vi "log analysis_gps.vi"() -> ()   [LabVIEW 2019] (continued)
03*697ae526\n\tsystem status\tnormal 2 28.100000 0 0\trobot status\t219.301877\t108.117218\t8.204700\t-1.556836\t0.092169\t-13.868102\t0.000000\t0.000000\n\t\n15:19:07.8\tlog_raw\tgps_raw\t#DUALANTENNAHEADINGA,USB3,0,49.0,FINESTEERING,2107,281965.800,02008000,d426,15824;SOL_COMPUTED,NARROW_FLOAT,-1.000000000,141.790161133,47.706295013,0.0,360.000000000,180.000000000,\"631T\",19,7,7,7,04,00,20,03*80dc72b9\n\tsystem status\tnormal 2 28.200000 0 0\trobot status\t219.302350\t108.113495\t8.203600\t-1.556726\t0.093605\t-13.864311\t0.000000\t0.000000\n\t\n15:19:08.3\tlog_raw\tgps_raw\t#DUALANTENNAHEADINGA,USB3,0,48.5,FINESTEERING,2107,281966.300,02008000,d426,15824;SOL_COMPUTED,NARROW_FLOAT,-1.000000000,166.037078857,-7.414306641,0.0,293.067352295,180.000000000,\"631T\",18,7,7,7,04,00,20,03*b88985fa\n\tsystem status\tnormal 2 28.200000 0 0\trobot status\t219.302993\t108.111164\t8.202900\t-1.556945\t0.093314\t-13.860391\t0.000000\t0.000000\n\t\n15:19:08.8\tlog_raw\tgps_raw\t#DUALANTENNAHEADINGA,USB3,0,48.5,FINESTEERING,2107,281966.800,02008000,d426,15824;SOL_COMPUTED,NARROW_FLOAT,-1.000000000,165.893447876,-6.919708252,0.0,296.453521729,180.000000000,\"631T\",17,7,7,7,04,00,20,03*8e2fbaf6\n\tsystem status\tnormal 2 28.100000 0 0\trobot status\t219.303827\t108.110162\t8.202400\t-1.557673\t0.092284\t-13.858493\t0.000000\t0.000000\n\t\n15:19:09.3\tlog_raw\tgps_raw\t#DUALANTENNAHEADINGA,USB3,0,48.5,FINESTEERING,2107,281967.300,02008000,d426,15824;SOL_COMPUTED,NARROW_FLOAT,-1.000000000,160.223464966,16.144151688,0.0,238.524597168,180.000000000,\"631T\",17,9,9,9,04,00,20,23*6b3012d0\n\tsystem status\tnormal 2 28.100000 0 0\trobot status\t219.306713\t108.109707\t8.201900\t-1.552890\t0.147275\t-13.759160\t0.122000\t-0.037000\n\t\n15:19:09.8\tlog_raw\tgps_raw\t#DUALANTENNAHEADINGA,USB3,0,48.5,FINESTEERING,2107,281967.800,02008000,d426,15824;SOL_COMPUTED,NARROW_FLOAT,-1.000000000,161.228576660,12.383532524,0.0,230.067184448,180.000000000,\"631T\",17,9,9,9,04,00,20,23*e747bf89\n\tsystem status\tnormal 2 28.100000 0 0\trobot status\t219.452339\t108.074928\t8.203100\t-1.465337\t0.190470\t-13.748043\t0.310000\t-0.019000\n\t\n15:19:10.3\tlog_raw\tgps_raw\t#DUALANTENNAHEADINGA,USB3,0,48.5,FINESTEERING,2107,281968.300,02000000,d426,15824;SOL_COMPUTED,NARROW_FLOAT,-1.000000000,166.146408081,14.704567909,0.0,156.659332275,180.000000000,\"631T\",17,9,9,9,04,00,20,23*68c6ea3a\n\tsystem status\tnormal 2 28.100000 0 0\trobot status\t219.578981\t108.043104\t8.204000\t-1.443728\t0.109997\t-13.833640\t0.283000\t-0.029000\n\t\n15:19:10.8\tlog_raw\tgps_raw\t#DUALANTENNAHEADINGA,USB3,0,48.5,FINESTEERING,2107,281968.800,02000000,d426,15824;SOL_COMPUTED,NARROW_FLOAT,-1.000000000,165.495330811,15.543543816,0.0,158.767318726,180.000000000,\"631T\",20,9,9,9,04,00,20,23*d314ab6c\n\tsystem status\tnormal 2 28.100000 0 0\trobot status\t219.724585\t108.004268\t8.205700\t-1.319380\t-0.022819\t-13.987268\t0.304000\t-0.003000\n\t\n15:19:11.3\tlog_raw\tgps_raw\t#DUALANTENNAHEADINGA,USB3,0,49.0,FINESTEERING,2107,281969.300,02000000,d426,15824;SOL_COMPUTED,NARROW_FLOAT,-1.000000000,139.943130493,-43.141418457,0.0,292.614349365,180.000000000,\"631T\",18,9,9,9,04,00,20,23*245444fd\n\tsystem status\tnormal 2 28.100000 0 0\trobot status\t219.855800\t107.968427\t8.207300\t-1.286734\t-0.015172\t-14.026863\t0.301000\t-0.006000\n\t\n15:19:11.8\tlog_raw\tgps_raw\t#DUALANTENNAHEADINGA,USB3,0,49.0,FINESTEERING,2107,281969.800,02000000,d426,15824;SOL_COMPUTED,NARROW_FLOAT,-1.000000000,140.197708130,-42.675354004,0.0,291.665954590,180.000000000,\"631T\",18,9,9,9,04,00,20,23*76897fdf\n\tsystem status\tnormal 2 28.100000 0 0\trobot status\t219.994546\t107.929885\t8.209200\t-1.297821\t0.001182\t-14.197346\t0.292000\t-0.016000\n\t\n15:19:12.3\tlog_raw\tgps_raw\t#DUALANTENNAHEADINGA,USB3,0,47.0,FINESTEERING,2107,281970.300,02000000,d426,15824;SOL_COMPUTED,NARROW_FLOAT,-1.000000000,136.818527222,-33.589324951,0.0,360.000000000,180.000000000,\"631T\",19,9,9,9,04,00,20,23*7b126b36\n\tsystem status\tnormal 2 28.100000 0 0\trobot status\t220.128217\t107.891100\t8.212500\t-1.413694\t0.161534\t-14.297386\t0.300000\t-0.004000\n\t\n15:19:12.8\tlog_raw\tgps_raw\t#DUALANTENNAHEADINGA,USB3,0,47.0,FINESTEERING,2107,281970.800,02000000,d426,15824;SOL_COMPUTED,NARROW_FLOAT,-1.000000000,136.650482178,-33.009735107,0.0,360.000000000,180.000000000,\"631T\",18,9,9,9,04,00,20,23*68bce87c\n\tsystem status\tnormal 2 28.100000 0 0\trobot status\t220.263771\t107.850315\t8.215700\t-1.551866\t0.293784\t-14.401574\t0.293000\t-0.008000\n\t\n15:19:13.3\tlog_raw\tgps_raw\t#DUALANTENNAHEADINGA,USB3,0,45.5,FINESTEERING,2107,281971.300,02000000,d426,15824;SOL_COMPUTED,NARROW_FLOAT,-1.000000000,137.123779297,-38.778259277,0.0,360.000000000,180.000000000,\"631T\",18,9,9,9,04,00,20,23*afd68441\n\tsystem status\tnormal 2 28.100000 0 0\trobot status\t220.401004\t107.805900\t8.218700\t-1.450367\t0.498611\t-14.556311\t0.301000\t-0.011000\n\t\n15:19:13.8\tlog_raw\tgps_raw\t#DUALANTENNAHEADINGA,USB3,0,45.5,FINESTEERING,2107,281971.800,02000000,d426,15824;SOL_COMPUTED,NARROW_FLOAT,-1.000000000,138.481918335,-40.903717041,0.0,360.000000000,180.000000000,\"631T\",17,7,7,7,04,00,20,03*998ba3b4\n\tsystem status\tnormal 2 28.100000 0 0\trobot status\t220.538888\t107.760543\t8.220800\t-1.387819\t0.562236\t-14.770983\t0.297000\t-0.058000\n\t\n15:19:14.3\tlog_raw\tgps_raw\t#DUALANTENNAHEADINGA,USB3,0,48.5,FINESTEERING,2107,281972.300,02000000,d426,15824;SOL_COMPUTED,NARROW_FLOAT,-1.000000000,122.800582886,-18.535125732,0.0,360.000000000,180.000000000,\"631T\",18,7,7,7,04,00,20,03*a3dfc53a\n\tsystem status\tnormal 2 28.100000 0 0\trobot status\t220.684115\t107.713725\t8.225400\t-1.489746\t0.729168\t-15.149259\t0.323000\t-0.019000\n\t\n15:19:14.8\tlog_raw\tgps_raw\t#DUALANTENNAHEADINGA,USB3,0,48.5,FINESTEERING,2107,281972.800,02000000,d426,15824;SOL_COMPUTED,NARROW_FLOAT,-1.000000000,124.024436951,-18.181030273,0.0,360.000000000,180.000000000,\"631T\",19,7,7,7,04,00,20,03*7aaae106\n\tsystem status\tnormal 2 28.000000 0 0\trobot status\t220.823247\t107.667621\t8.231100\t-1.707730\t0.719198\t-15.929117\t0.256000\t-0.109000\n\t\n15:19:15.3\tlog_raw\tgps_raw\t#DUALANTENNAHEADINGA,USB3,0,47.5,FINESTEERING,2107,281973.300,02000000,d426,15824;SOL_COMPUTED,NARROW_FLOAT,-1.000000000,122.042884827,-22.737487793,0.0,360.000000000,180.000000000,\"631T\",19,7,7,7,04,00,20,03*1f55fb10\n\tsystem status\tnormal 2 28.000000 0 0\trobot status\t220.956067\t107.616714\t8.234300\t-1.546838\t0.621611\t-17.048894\t0.328000\t-0.004000\n\t\n15:19:15.8\tlog_raw\tgps_raw\t#DUALANTENNAHEADINGA,USB3,0,47.5,FINESTEERING,2107,281973.800,02000000,d426,15824;SOL_COMPUTED,NARROW_FLOAT,-1.000000000,123.718307495,-22.855773926,0.0,360.000000000,180.000000000,\"631T\",19,7,7,7,04,00,20,03*d5b1223e\n\tsystem status\tnormal 2 27.800000 0 0\trobot status\t221.089499\t107.561166\t8.235900\t-1.404373\t0.484391\t-18.472087\t0.229000\t-0.159000\n\t\n15:19:16.3\tlog_raw\tgps_raw\t#DUALANTENNAHEADINGA,USB3,0,47.5,FINESTEERING,2107,281974.300,02000000,d426,15824;SOL_COMPUTED,NARROW_FLOAT,-1.000000000,126.303939819,-25.588958740,0.0,360.000000000,180.000000000,\"631T\",20,7,7,7,04,00,20,03*39a380db\n\tsystem status\tnormal 2 27.800000 0 0\trobot status\t221.221746\t107.503167\t8.238200\t-1.480054\t0.670255\t-19.868861\t0.268000\t-0.096000\n\t\n15:19:16.8\tlog_raw\tgps_raw\t\tsystem status\tnormal 2 27.800000 0 0\trobot status\t221.353565\t107.442341\t8.242100\t-1.646339\t0.593532\t-21.133921\t0.306000\t-0.008000\n\t\n15:19:17.3\tlog_raw\tgps_raw\t\tsystem status\tnormal 2 28.000000 0 0\trobot status\t221.483986\t107.376940\t8.246600\t-1.582498\t0.515204\t-22.081277\t0.288000\t-0.060000\n\t\n15:19:17.8\tlog_raw\tgps_raw\t\tsystem status\tnormal 2 28.000000 0 0\trobot status\t221.610837\t107.309899\t8.249600\t-1.462249\t0.554475\t-22.719176\t0.412000\t0.141000\n\t\n15:19:18.3\tlog_raw\tgps_raw\t\tsystem status\tnormal 2 28.100000 0 0\trobot status\t221.736004\t107.242196\t8.251300\t-1.432747\t0.573608\t-23.074714\t0.316000\t0.037000\n\t\n15:19:18.8\tlog_raw\tgps_raw\t\tsystem status\tnormal 2 28.100000 0 0\trobot status\t221.859914\t107.174246\t8.252600\t-1.427237\t0.406480\t-23.239314\t0.289000\t0.008000\n\t\n15:19:19.3\tlog_raw\tgps_raw\t#INSPVAXA,USB3,0,49.5,FINESTEERING,2107,281977.350,02008000,471d,15824;INS_ALIGNMENT_COMPLETE,INS_RTKFIXED,37.37109525402,126.72334121062,8.2543,22.3000,-0.1170,0.2421,0.0133,-1.435832187,0.337185774,113.410271664,0.3981,0.2933,0.5166,0.1081,0.0923,0.0755,0.1541,0.1553,4.9775,0f000001,0*5c2d119f\n\tsystem status\tnormal 2 28.100000 0 0\trobot status\t221.986722\t107.103576\t8.254300\t-1.435832\t0.337186\t-23.410272\t0.294000\t0.028000\n\t\n15:19:19.8\tlog_raw\tgps_raw\t\tsystem status\tnormal 2 28.100000 0 0\trobot status\t222.097089\t107.042706\t8.257000\t-1.370753\t0.338842\t-23.399913\t0.298000\t0.032000\n\t\n15:19:20.3\tlog_raw\tgps_raw\t\tsystem status\tnormal 2 28.100000 0 0\trobot status\t222.231985\t106.969531\t8.259800\t-1.288256\t0.476149\t-23.360701\t0.319000\t0.022000\n\t\n15:19:20.8\tlog_raw\tgps_raw\t#DUALANTENNAHEADINGA,USB3,0,47.5,FINESTEERING,2107,281978.800,02008000,d426,15824;SOL_COMPUTED,NARROW_FLOAT,-1.000000000,98.850494385,15.051933289,0.0,360.000000000,180.000000000,\"631T\",20,7,7,7,04,00,20,03*20b61e65\n\tsystem status\tnormal 2 28.000000 0 0\trobot status\t222.361467\t106.898858\t8.261700\t-1.138019\t0.411063\t-23.031329\t0.236000\t0.133000\n\t\n15:19:21.3\tlog_raw\tgps_raw\t#INSPVAXA,USB3,0,49.0,FINESTEERING,2107,281979.350,02008000,471d,15824;INS_ALIGNMENT_COMPLETE,INS_RTKFIXED,37.37109277757,126.72334695019,8.2625,22.3000,-0.1363,0.2541,0.0099,-1.083954396,0.543239164,111.989343761,0.3985,0.2934,0.5159,0.1083,0.0925,0.0755,0.1539,0.1552,4.9769,0f000001,0*5af8ae3d\n\tsystem status\tnormal 2 27.900000 0 0\trobot status\t222.495124\t106.828715\t8.262500\t-1.083954\t0.543239\t-21.989344\t0.244000\t0.133000\n\t\n15:19:21.8\tlog_raw\tgps_raw\t#INSPVAXA,USB3,0,49.0,FINESTEERING,2107,281979.850,02008000,471d,15824;INS_ALIGNMENT_COMPLETE,INS_RTKFIXED,37.37109223488,126.72334834985,8.2645,22.3000,-0.1140,0.2510,0.0288,-1.130767744,0.597027739,110.592195970,0.3985,0.2934,0.5159,0.1083,0.0925,0.0755,0.1539,0.1552,4.9769,0f000001,0*c15e5176\n\tsystem status\tnormal 2 27.700000 0 0\trobot status\t222.619104\t106.768481\t8.264500\t-1.130768\t0.597028\t-20.592196\t0.292000\t0.067000\n\t\n15:19:22.3\tlog_raw\tgps_raw\t#INSPVAXA,USB3,0,47.5,FINESTEERING,2107,281980.350,02008000,471d,15824;INS_ALIGNMENT_COMPLETE,INS_RTKFIXED,37.37109170650,126.72334980236,8.2673,22.3000,-0.1001,0.2682,0.0069,-1.052775412,0.394834904,108.778696674,0.3992,0.2936,0.5159,0.1082,0.0924,0.0755,0.1537,0.1552,4.9781,0f000001,0*7c12e27f\n\tsystem status\tnormal 2 27.500000 0 0\trobot status\t222.747765\t106.709836\t8.267300\t-1.052775\t0.394835\t-18.778697\t0.298000\t0.063000\n\t\n15:19:22.8\tlog_raw\tgps_raw\t\tsystem status\tnormal 2 27.500000 0 0\trobot status\t222.863745\t106.660014\t8.268600\t-0.838461\t0.276001\t-16.977261\t0.297000\t0.053000\n\t\n15:19:23.3\tlog_raw\tgps_raw\t\tsystem status\tnormal 2 27.600000 4 0\trobot status\t222.994027\t106.612485\t8.270800\t-0.856834\t0.314980\t-15.099494\t0.306000\t0.063000\n\t\n15:19:23.8\tlog_raw\tgps_raw\t#DUALANTENNAHEADINGA,USB3,0,47.5,FINESTEERING,2107,281981.800,02000000,d426,15824;SOL_COMPUTED,NARROW_FLOAT,-1.000000000,85.660850525,58.330966949,0.0,360.000000000,180.000000000,\"631T\",21,7,7,7,04,00,20,03*4d1d89aa\n\tsystem status\tnormal 2 27.600000 4 0\trobot status\t223.126606\t106.570431\t8.273400\t-0.931607\t0.502901\t-13.314554\t0.308000\t0.043000\n\t\n15:19:24.3\tlog_raw\tgps_raw\t#DUALANTENNAHEADINGA,USB3,0,50.0,FINESTEERING,2107,281982.300,02000000,d426,15824;SOL_COMPUTED,NARROW_FLOAT,-1.000000000,91.491950989,60.466197968,0.0,360.000000000,180.000000000,\"631T\",20,7,7,7,04,00,20,03*c36635f4\n\tsystem status\tnormal 2 27.700000 0 0\trobot status\t223.261861\t106.529900\t8.275300\t-0.949553\t0.583973\t-11.945884\t0.297000\t0.040000\n\t\n15:19:24.8\tlog_raw\tgps_raw\t#INSPVAXA,USB3,0,50.0,FINESTEERING,2107,281982.850,02000000,471d,15824;INS_ALIGNMENT_COMPLETE,INS_RTKFIXED,37.37108972334,126.72335727408,8.2765,22.3000,-0.0719,0.2745,0.0019,-0.882780999,0.621145349,100.706035847,0.4014,0.2941,0.5170,0.1080,0.0922,0.0756,0.1534,0.1551,4.9808,0f000001,0*8125501e\n\tsystem status\tnormal 2 27.800000 0 0\trobot status\t223.409597\t106.489718\t8.276500\t-0.882781\t0.621145\t-10.706036\t0.293000\t0.023000\n\t\n15:19:25.3\tlog_raw\tgps_raw\t#INSPVAXA,USB3,0,50.0,FINESTEERING,2107,281983.350,02000000,471d,15824;INS_ALIGNMENT_COMPLETE,INS_RTKFIXED,37.37108941060,126.72335884904,8.2775,22.3000,-0.0682,0.2732,0.0044,-0.923445241,0.570606405,99.817736396,0.4009,0.2937,0.5167,0.1077,0.0921,0.0755,0.1533,0.1550,4.9813,0f000001,0*fb321f29\n\tsystem status\tnormal 2 27.800000 0 0\trobot status\t223.549105\t106.455005\t8.277500\t-0.923445\t0.570606\t-9.817736\t0.249000\t0.097000\n\t\n15:19:25.8\tlog_raw\tgps_raw\t#DUALANTENNAHEADINGA,USB3,0,50.0,FINESTEERING,2107,281983.800,02000000,d426,15824;SOL_COMPUTED,NARROW_FLOAT,-1.000000000,171.677200317,69.382904053,0.0,261.160797119,118.765472412,\"631T\",16,7,7,7,04,00,20,03*68664d6e\n\tsystem status\tnormal 2 27.900000 0 0\trobot status\t223.673813\t106.423577\t8.278600\t-0.753862\t0.396065\t-9.286254\t0.221000\t0.059000\n\t\n15:19:26.3\tlog_raw\tgps_raw\t\tsystem status\tnormal 2 28.100000 0 0\trobot status\t223.691032\t106.410286\t8.277000\t-0.784481\t0.395097\t-9.504168\t0.001000\t0.000000\n\t\n15:19:26.8\tlog_raw\tgps_raw\t#DUALANTENNAHEADINGA,USB3,0,49.0,FINESTEERING,2107,281984.800,02000000,d426,15824;SOL_COMPUTED,NARROW_FLOAT,-1.000000000,180.068710327,69.173255920,0.0,191.709030151,111.731857300,\"631T\",18,7,7,7,04,00,20,03*3faf2cde\n\tsystem status\tnormal 2 28.100000 0 0\trobot status\t223.690316\t106.399747\t8.275200\t-0.784448\t0.393746\t-9.515483\t0.000000\t0.000000\n\t\n15:19:27.3\tlog_raw\tgps_raw\t#INSPVAXA,USB3,0,51.5,FINESTEERING,2107,281985.350,02000000,471d,15824;INS_ALIGNMENT_COMPLETE,INS_RTKFIXED,37.37108883978,126.72336045763,8.2740,22.3000,-0.0197,0.0054,0.0046,-0.783405555,0.390647361,99.517937429,0.4021,0.2930,0.5155,0.1100,0.0923,0.0753,0.1532,0.1549,4.9767,0f000001,0*248bca7d\n\tsystem status\tnormal 2 28.100000 0 0\trobot status\t223.691591\t106.391649\t8.274000\t-0.783406\t0.390647\t-9.517937\t0.000000\t0.000000\n\t\n15:19:27.8\tlog_raw\tgps_raw\t#INSPVAXA,USB3,0,51.5,FINESTEERING,2107,281985.850,02000000,471d,15824;INS_ALIGNMENT_COMPLETE,INS_RTKFIXED,37.37108879564,126.72336048903,8.2732,22.3000,-0.0176,0.0072,0.0041,-0.785106816,0.393235507,99.515755196,0.4021,0.2930,0.5155,0.1100,0.0923,0.0753,0.1532,0.1549,4.9767,0f000001,0*274b58cf\n\tsystem status\tnormal 2 28.100000 0 0\trobot status\t223.694372\t106.386750\t8.273200\t-0.785107\t0.393236\t-9.515755\t0.000000\t0.000000\n\t\n15:19:28.3\tlog_raw\tgps_raw\t#INSPVAXA,USB3,0,48.0,FINESTEERING,2107,281986.350,02000000,471d,15824;INS_ALIGNMENT_COMPLETE,INS_RTKFIXED,37.37108876739,126.72336052169,8.2716,22.3000,-0.0165,0.0095,0.0036,-0.784401118,0.395223207,99.515202134,0.4035,0.2929,0.5152,0.1096,0.0926,0.0753,0.1533,0.1548,4.9684,0f000001,0*a346e64c\n\tsystem status\tnormal 2 28.100000 0 0\trobot status\t223.697265\t106.383614\t8.271600\t-0.784401\t0.395223\t-9.515202\t0.000000\t0.000000\n\t\n15:19:28.8\tlog_raw\tgps_raw\t#INSPVAXA,USB3,0,48.0,FINESTEERING,2107,281986.850,02000000,471d,15824;INS_ALIGNMENT_COMPLETE,INS_RTKFIXED,37.37108874345,126.72336056234,8.2697,22.3000,-0.0165,0.0121,0.0038,-0.783492402,0.394489755,99.515268090,0.4035,0.2929,0.5152,0.1096,0.0926,0.0753,0.1533,0.1548,4.9684,0f000001,0*d15eefc4\n\tsystem status\tnormal 2 28.100000 0 0\trobot status\t223.700866\t106.380957\t8.269700\t-0.783492\t0.394490\t-9.515268\t0.000000\t0.000000\n\t\n15:19:29.3\tlog_raw\tgps_raw\t\tsystem status\tnormal 2 28.000000 0 0\trobot status\t223.744232\t106.373691\t8.270100\t-0.798843\t0.520000\t-9.359082\t0.297000\t-0.003000\n\t\n15:19:29.8\tlog_raw\tgps_raw\t\tsystem status\tnormal 2 28.100000 0 0\trobot status\t223.909115\t106.346672\t8.272000\t-0.747510\t0.256715\t-9.615742\t0.328000\t-0.055000\n\t\n15:19:30.3\tlog_raw\tgps_raw\t\tsystem status\tnormal 2 28.100000 0 0\trobot status\t224.051089\t106.323073\t8.274200\t-0.894303\t0.217307\t-9.628486\t0.311000\t-0.011000\n\t\n15:19:30.8\tlog_raw\tgps_raw\t#INSPVAXA,USB3,0,47.5,FINESTEERING,2107,281988.850,02000000,471d,15824;INS_ALIGNMENT_COMPLETE,INS_RTKFIXED,37.37108797326,126.72336627998,8.2767,22.3000,-0.0630,0.2990,0.0131,-1.082198945,0.183813421,99.716659847,0.4039,0.2931,0.5146,0.1091,0.0928,0.0753,0.1533,0.1544,4.9498,0f000001,0*73d74fed\n\tsystem status\tnormal 2 28.100000 0 0\trobot status\t224.207325\t106.295465\t8.276700\t-1.082199\t0.183813\t-9.716660\t0.302000\t-0.009000\n\t\n15:19:31.3\tlog_raw\tgps_raw\t#INSPVAXA,USB3,0,47.5,FINESTEERING,2107,281989.350,02000000,471d,15824;INS_ALIGNMENT_COMPLETE,INS_RTKFIXED,37.37108771760,126.72336784946,8.2786,22.3000,-0.0596,0.2938,0.0092,-0.873489656,0.138919963,99.763055093,0.4016,0.2938,0.5156,0.1102,0.0931,0.0754,0.1533,0.1542,4.9496,0f000001,0*cc44b012\n\tsystem status\tnormal 2 28.100000 0 0\trobot status\t224.346347\t106.267087\t8.278600\t-0.873490\t0.138920\t-9.763055\t0.292000\t0.011000\n\t\n15:19:31.8\tlog_raw\tgps_raw\t\tsystem status\tnormal 2 28.100000 0 0\trobot status\t224.485443\t106.239017\t8.280100\t-0.782767\t-0.017640\t-9.679057\t0.297000\t0.017000\n\t\n15:19:32.3\tlog_raw\tgps_raw\t\tsystem status\tnormal 2 28.000000 0 0\trobot status\t224.626651\t106.210499\t8.281900\t-0.769512\t0.068077\t-9.236097\t0.360000\t-0.076000\n\t\n15:19:32.8\tlog_raw\tgps_raw\t#INSPVAXA,USB3,0,48.0,FINESTEERING,2107,281990.850,02000000,471d,15824;INS_ALIGNMENT_COMPLETE,INS_RTKFIXED,37.37108694002,126.72337277307,8.2855,22.3000,-0.0481,0.3030,0.0049,-0.965496149,0.214981023,98.709278858,0.4041,0.2964,0.5214,0.1116,0.0937,0.0758,0.1533,0.1541,4.9510,0f000001,0*3e871dfa\n\tsystem status\tnormal 2 28.000000 0 0\trobot status\t224.782473\t106.180775\t8.285500\t-0.965496\t0.214981\t-8.709279\t0.336000\t-0.030000\n\t\n15:19:33.3\tlog_raw\tgps_raw\t#INSPVAXA,USB3,0,49.5,FINESTEERING,2107,281991.350,02000000,471d,15824;INS_ALIGNMENT_COMPLETE,INS_RTKFIXED,37.37108669886,126.72337439108,8.2873,22.3000,-0.0502,0.3004,0.0017,-1.174650007,0.215279567,98.185602057,0.4065,0.2980,0.5270,0.1121,0.0939,0.0762,0.1533,0.1539,4.9506,0f000001,0*29bf6a14\n\tsystem status\tnormal 2 28.000000 0 0\trobot status\t224.925793\t106.154006\t8.287300\t-1.174650\t0.215280\t-8.185602\t0.248000\t0.089000\n\t\n15:19:33.8\tlog_raw\tgps_raw\t\tsystem status\tnormal 2 28.000000 0 0\trobot status\t225.055464\t106.128832\t8.288900\t-1.106111\t0.185902\t-7.711529\t0.340000\t-0.056000\n\t\n15:19:34.3\tlog_raw\tgps_raw\t#INSPVAXA,USB3,0,48.5,FINESTEERING,2107,281992.350,02008000,471d,15824;INS_ALIGNMENT_COMPLETE,INS_RTKFIXED,37.37108621097,126.72337762308,8.2906,22.3000,-0.0509,0.3067,0.0077,-1.111919380,0.301360235,97.469482841,0.4135,0.2993,0.5341,0.1130,0.0941,0.0766,0.1532,0.1538,4.9480,0f000001,0*f7c4fc4c\n\tsystem status\tnormal 2 28.000000 0 0\trobot status\t225.212079\t106.099851\t8.290600\t-1.111919\t0.301360\t-7.469483\t0.444000\t-0.212000\n\t\n15:19:34.8\tlog_raw\tgps_raw\t#INSPVAXA,USB3,0,48.5,FINESTEERING,2107,281992.850,02008000,471d,15824;INS_ALIGNMENT_COMPLETE,INS_RTKFIXED,37.37108597752,126.72337923306,8.2930,22.3000,-0.0486,0.3061,0.0133,-1.174980887,0.150326123,97.387759398,0.4135,0.2993,0.5341,0.1130,0.0941,0.0766,0.1532,0.1538,4.9480,0f000001,0*c1faa1b5\n\tsystem status\tnormal 2 28.000000 0 0\trobot status\t225.354688\t106.073937\t8.293000\t-1.174981\t0.150326\t-7.387759\t0.359000\t-0.095000\n\t\n15:19:35.3\tlog_raw\tgps_raw\t#INSPVAXA,USB3,0,46.0,FINESTEERING,2107,281993.350,02008000,471d,15824;INS_ALIGNMENT_COMPLETE,INS_RTKFIXED,37.37108573998,126.72338082832,8.2949,22.3000,-0.0500,0.2978,0.0061,-1.421543632,0.145972145,97.447075083,0.4166,0.2999,0.5394,0.1132,0.0941,0.0768,0.1531,0.1535,4.9437,0f000001,0*17ed31ac\n\tsystem status\tnormal 2 28.100000 0 0\trobot status\t225.495993\t106.047570\t8.294900\t-1.421544\t0.145972\t-7.447075\t0.251000\t0.057000\n\t\n15:19:35.8\tlog_raw\tgps_raw\t#INSPVAXA,USB3,0,46.0,FINESTEERING,2107,281993.850,02008000,471d,15824;INS_ALIGNMENT_COMPLETE,INS_RTKFIXED,37.37108548434,126.72338234457,8.2959,22.3000,-0.0500,0.2833,0.0078,-1.457872405,0.272327462,97.575825981,0.4166,0.2999,0.5394,0.1132,0.0941,0.0768,0.1531,0.1535,4.9437,0f000001,0*5caa60c3\n\tsystem status\tnormal 2 28.100000 0 0\trobot status\t225.630300\t106.019194\t8.295900\t-1.457872\t0.272327\t-7.575826\t0.294000\t-0.026000\n\t\n15:19:36.3\tlog_raw\tgps_raw\t\tsystem status\tnormal 2 28.100000 0 0\trobot status\t225.748467\t105.992775\t8.298600\t-1.403323\t0.357170\t-7.675488\t0.298000\t-0.031000\n\t\n15:19:36.8\tlog_raw\tgps_raw\t#INSPVAXA,USB3,0,49.0,FINESTEERING,2107,281994.850,02008000,471d,15824;INS_ALIGNMENT_COMPLETE,INS_RTKFIXED,37.37108494308,126.72338542204,8.3016,22.3000,-0.0524,0.2963,0.0111,-1.327091398,0.262905229,97.908015700,0.4162,0.2999,0.5423,0.1120,0.0939,0.0768,0.1530,0.1531,4.9380,0f000001,0*42f9b06f\n\tsystem status\tnormal 2 28.100000 0 0\trobot status\t225.902898\t105.959116\t8.301600\t-1.327091\t0.262905\t-7.908016\t0.294000\t-0.034000\n\t\n15:19:37.3\tlog_raw\tgps_raw\t#INSPVAXA,USB3,0,47.5,FINESTEERING,2107,281995.350,02008000,471d,15824;INS_ALIGNMENT_COMPLETE,INS_RTKFIXED,37.37108466032,126.72338706837,8.3039,22.3000,-0.0576,0.3333,-0.0065,-1.460342907,0.308573578,98.178770776,0.4137,0.2991,0.5422,0.1112,0.0936,0.0766,0.1529,0.1527,4.9332,0f000001,0*ae64a2a4\n\tsystem status\tnormal 2 28.100000 0 0\trobot status\t226.048727\t105.927730\t8.303900\t-1.460343\t0.308574\t-8.178771\t0.301000\t-0.034000\n\t\n15:19:37.8\tlog_raw\tgps_raw\t#INSPVAXA,USB3,0,47.5,FINESTEERING,2107,281995.850,02008000,471d,15824;INS_ALIGNMENT_COMPLETE,INS_RTKFIXED,37.37108438124,126.72338871075,8.3072,22.3000,-0.0531,0.3233,-0.0006,-1.819145416,0.336322767,98.552237530,0.4137,0.2991,0.5422,0.1112,0.0936,0.0766,0.1529,0.1527,4.9332,0f000001,0*cbb88409\n\tsystem status\tnormal 2 28.100000 0 0\trobot status\t226.194206\t105.896752\t8.307200\t-1.819145\t0.336323\t-8.552238\t0.312000\t-0.021000\n\t\n15:19:38.3\tlog_raw\tgps_raw\t#INSPVAXA,USB3,0,47.5,FINESTEERING,2107,281996.350,02000000,471d,15824;INS_ALIGNMENT_COMPLETE,INS_RTKFIXED,37.37108408170,126.72339032288,8.3123,22.3000,-0.0750,0.3139,0.0177,-1.695760628,0.287982482,99.034005489,0.4135,0.2988,0.5426,0.1109,0.0935,0.0765,0.1528,0.1525,4.9294,0f000001,0*c8ba75d6\n\tsystem status\tnormal 2 28.100000 0 0\trobot status\t226.337006\t105.863504\t8.312300\t-1.695761\t0.287982\t-9.034005\t0.263000\t-0.087000\n\t\n15:19:38.8\tlog_raw\tgps_raw\t#INSPVAXA,USB3,0,47.5,FINESTEERING,2107,281996.850,02000000,471d,15824;INS_ALIGNMENT_COMPLETE,INS_RTKFIXED,37.37108376936,126.72339189832,8.3173,22.3000,-0.0870,0.3015,0.0104,-1.544598209,0.423694709,99.865488428,0.4135,0.2988,0.5426,0.1109,0.0935,0.0765,0.1528,0.1525,4.9294,0f000001,0*decac9b0\n\tsystem status\tnormal 2 28.000000 0 0\trobot status\t226.476556\t105.828835\t8.317300\t-1.544598\t0.423695\t-9.865488\t0.314000\t-0.012000\n\t\n15:19:39.3\tlog_raw\tgps_raw\t#INSPVAXA,USB3,0,47.0,FINESTEERING,2107,281997.350,02000000,471d,15824;INS_ALIGNMENT_COMPLETE,INS_RTKFIXED,37.37108342179,126.72339342311,8.3197,22.3000,-0.0655,0.2686,0.0098,-1.474135417,0.714052944,100.935237660,0.4109,0.2981,0.5411,0.1099,0.0931,0.0764,0.1526,0.1523,4.9264,0f000001,0*027bf543\n\tsystem status\tnormal 2 28.000000 0 0\trobot status\t226.611619\t105.790257\t8.319700\t-1.474135\t0.714053\t-10.935238\t0.298000\t-0.044000\n\t\n15:19:39.8\tlog_raw\tgps_raw\t#INSPVAXA,USB3,0,47.0,FINESTEERING,2107,281997.850,02000000,471d,15824;INS_ALIGNMENT_COMPLETE,INS_RTKFIXED,37.37108303856,126.72339495769,8.3212,22.3000,-0.0845,0.2926,0.0185,-1.495781982,0.741465354,102.154050788,0.4109,0.2981,0.5411,0.1099,0.0931,0.0764,0.1526,0.1523,4.9264,0f000001,0*92cd812c\n\tsystem status\tnormal 2 27.800000 0 0\trobot status\t226.747550\t105.747720\t8.321200\t-1.495782\t0.741465\t-12.154051\t0.325000\t-0.013000\n\t\n15:19:40.3\tlog_raw\tgps_raw\t#DUALANTENNAHEADINGA,USB3,0,46.5,FINESTEERING,2107,281998.300,02000000,d426,15824;SOL_COMPUTED,NARROW_FLOAT,-1.000000000,172.084686279,54.228965759,0.0,275.366882324,180.000000000,\"631T\",18,9,9,9,04,00,20,23*6c4f8940\n\tsystem status\tnormal 2 27.800000 0 0\trobot status\t226.869310\t105.708063\t8.323600\t-1.489847\t0.680798\t-13.305228\t0.285000\t-0.048000\n\t\n15:19:40.8\tlog_raw\tgps_raw\t#INSPVAXA,USB3,0,46.5,FINESTEERING,2107,281998.850,02000000,471d,15824;INS_ALIGNMENT_COMPLETE,INS_RTKFIXED,37.37108222334,126.72339800305,8.3261,22.3000,-0.1005,0.2888,0.0175,-1.549699637,0.826090686,104.570528927,0.4090,0.2977,0.5394,0.1094,0.0929,0.0762,0.1525,0.1522,4.9251,0f000001,0*19ed46e2\n\tsystem status\tnormal 2 27.900000 0 0\trobot status\t227.017303\t105.657236\t8.326100\t-1.549700\t0.826091\t-14.570529\t0.291000\t-0.041000\n\t\n15:19:41.3\tlog_raw\tgps_raw\t#INSPVAXA,USB3,0,46.5,FINESTEERING,2107,281999.350,02000000,471d,15824;INS_ALIGNMENT_COMPLETE,INS_RTKFIXED,37.37108175635,126.72339952041,8.3297,22.3000,-0.1125,0.3020,0.0389,-1.388953063,0.939960250,105.504121807,0.4075,0.2973,0.5375,0.1091,0.0928,0.0761,0.1524,0.1521,4.9251,0f000001,0*0f043892\n\tsystem status\tnormal 2 27.900000 0 0\trobot status\t227.151708\t105.605404\t8.329700\t-1.388953\t0.939960\t-15.504122\t0.320000\t0.005000\n\t\n15:19:41.8\tlog_raw\tgps_raw\t#INSPVAXA,USB3,0,46.5,FINESTEERING,2107,281999.850,02000000,471d,15824;INS_ALIGNMENT_COMPLETE,INS_RTKFIXED,37.37108126318,126.72340101598,8.3324,22.3000,-0.1208,0.2855,0.0176,-1.235609650,1.001617450,106.317928452,0.4075,0.2973,0.5375,0.1091,0.0928,0.0761,0.1524,0.1521,4.9251,0f000001,0*a366704e\n\tsystem status\tnormal 2 28.000000 0 0\trobot status\t227.284183\t105.550666\t8.332400\t-1.235610\t1.001617\t-16.317928\t0.353000\t0.073000\n\t\n15:19:42.3\tlog_raw\tgps_raw\t#INSPVAXA,USB3,0,45.5,FINESTEERING,2107,282000.350,02000000,471d,15824;INS_ALIGNMENT_COMPLETE,INS_RTKFIXED,37.37108078810,126.72340249141,8.3350,22.3000,-0.1085,0.2765,0.0052,-1.369966017,1.132397768,106.939829870,0.4067,0.2969,0.5359,0.1090,0.0927,0.0761,0.1523,0.1521,4.9261,0f000001,0*76e4d7c9\n\tsystem status\tnormal 2 28.000000 0 0\trobot status\t227.414874\t105.497936\t8.335000\t-1.369966\t1.132398\t-16.939830\t0.348000\t0.059000\n\t\n15:19:42.8\tlog_raw\tgps_raw\t#INSPVAXA,USB3,0,45.5,FINESTEERING,2107,282000.850,02000000,471d,15824;INS_ALIGNMENT_COMPLETE,INS_RTKFIXED,37.37108030098,126.72340396380,8.3376,22.3000,-0.1078,0.2732,0.0027,-1.376343983,1.101027936,107.303720735,0.4067,0.2969,0.5359,0.1090,0.0927,0.0761,0.1523,0.1521,4.9261,0f000001,0*d0ca4e8b\n\tsystem status\tnormal 2 28.000000 0 0\trobot status\t227.545296\t105.443869\t8.337600\t-1.376344\t1.101028\t-17.303721\t0.357000\t0.093000\n\t\n15:19:43.3\tlog_raw\tgps_raw\t#INSPVAXA,USB3,0,48.0,FINESTEERING,2107,282001.350,02000000,471d,15824;INS_ALIGNMENT_COMPLETE,INS_RTKFIXED,37.37107981419,126.72340544381,8.3410,22.3000,-0.1015,0.2654,0.0098,-1.448342313,0.934631006,107.625890193,0.4067,0.2967,0.5346,0.1090,0.0928,0.0761,0.1522,0.1521,4.9276,0f000001,0*0452f07a\n\tsystem status\tnormal 2 28.100000 0 0\trobot status\t227.676393\t105.389840\t8.341000\t-1.448342\t0.934631\t-17.625890\t0.248000\t-0.063000\n\t\n15:19:43.8\tlog_raw\tgps_raw\t#INSPVAXA,USB3,0,48.0,FINESTEERING,2107,282001.850,02000000,471d,15824;INS_ALIGNMENT_COMPLETE,INS_RTKFIXED,37.37107932053,126.72340689230,8.3455,22.3000,-0.1081,0.2753,0.0156,-1.395073835,0.867862564,107.855111716,0.4067,0.2967,0.5346,0.1090,0.0928,0.0761,0.1522,0.1521,4.9276,0f000001,0*57502385\n\tsystem status\tnormal 2 28.100000 0 0\trobot status\t227.804698\t105.335047\t8.345500\t-1.395074\t0.867863\t-17.855112\t0.298000\t0.008000\n\t\n15:19:44.3\tlog_raw\tgps_raw\t\tsystem status\tnormal 2 28.100000 0 0\trobot status\t227.927954\t105.281998\t8.349000\t-1.240339\t0.748204\t-18.058239\t0.295000\t0.023000\n\t\n15:19:44.8\tlog_raw\tgps_raw\t\tsystem status\tnormal 2 28.100000 0 0\trobot status\t228.055523\t105.229241\t8.352400\t-1.309413\t0.605958\t-18.159902\t0.298000\t0.016000\n\t\n15:19:45.3\tlog_raw\tgps_raw\t#INSPVAXA,USB3,0,47.5,FINESTEERING,2107,282003.350,02000000,471d,15824;INS_ALIGNMENT_COMPLETE,INS_RTKFIXED,37.37107789784,126.72341117734,8.3560,22.3000,-0.1094,0.2769,0.0199,-1.466008388,0.636532591,108.200024976,0.4065,0.2960,0.5312,0.1093,0.0930,0.0760,0.1520,0.1521,4.9306,0f000001,0*2f9a30b4\n\tsystem status\tnormal 2 28.100000 0 0\trobot status\t228.184260\t105.177140\t8.356000\t-1.466008\t0.636533\t-18.200025\t0.298000\t0.029000\n\t\n15:19:45.8\tlog_raw\tgps_raw\t#INSPVAXA,USB3,0,47.5,FINESTEERING,2107,282003.850,02000000,471d,15824;INS_ALIGNMENT_COMPLETE,INS_RTKFIXED,37.37107739435,126.72341272898,8.3600,22.3000,-0.1006,0.2711,0.0114,-1.521008315,0.580444752,108.231718498,0.4065,0.2960,0.5312,0.1093,0.0930,0.0760,0.1520,0.1521,4.9306,0f000001,0*1b9fd745\n\tsystem status\tnormal 2 28.100000 0 0\trobot status\t228.321702\t105.121257\t8.360000\t-1.521008\t0.580445\t-18.231718\t0.296000\t0.025000\n\t\n15:19:46.3\tlog_raw\tgps_raw\t#INSPVAXA,USB3,0,50.0,FINESTEERING,2107,282004.350,02000000,471d,15824;INS_ALIGNMENT_COMPLETE,INS_RTKFIXED,37.37107686919,126.72341426546,8.3651,22.3000,-0.1209,0.2828,0.0059,-1.390875360,0.569748446,108.156890117,0.4068,0.2963,0.5308,0.1095,0.0933,0.0761,0.1519,0.1521,4.9320,0f000001,0*3c184099\n\tsystem status\tnormal 2 28.100000 0 0\trobot status\t228.457801\t105.062969\t8.365100\t-1.390875\t0.569748\t-18.156890\t0.313000\t0.022000\n\t\n15:19:46.8\tlog_raw\tgps_raw\t\tsystem status\tnormal 2 28.000000 0 0\trobot status\t228.586579\t105.005917\t8.370800\t-1.203332\t0.754103\t-17.940693\t0.298000\t0.017000\n\t\n15:19:47.3\tlog_raw\tgps_raw\t\tsystem status\tnormal 2 28.000000 0 0\trobot status\t228.718735\t104.952851\t8.376100\t-1.401587\t0.653594\t-17.475054\t0.249000\t0.095000\n\t\n15:19:47.8\tlog_raw\tgps_raw\t#INSPVAXA,USB3,0,51.0,FINESTEERING,2107,282005.850,02000000,471d,15824;INS_ALIGNMENT_COMPLETE,INS_RTKFIXED,37.37107540800,126.72341870261,8.3803,22.3000,-0.1004,0.2666,0.0170,-1.392102628,0.780129510,106.805722227,0.4082,0.2971,0.5322,0.1099,0.0935,0.0762,0.1518,0.1521,4.9335,0f000001,0*c4f2d669\n\tsystem status\tnormal 2 27.900000 0 0\trobot status\t228.850836\t104.900788\t8.380300\t-1.392103\t0.780130\t-16.805722\t0.259000\t0.094000\n\t\n15:19:48.3\tlog_raw\tgps_raw\t#INSPVAXA,USB3,0,50.5,FINESTEERING,2107,282006.350,02000000,471d,15824;INS_ALIGNMENT_COMPLETE,INS_RTKFIXED,37.37107495980,126.72342017770,8.3861,22.3000,-0.1091,0.2763,0.0150,-1.313432371,0.996573808,106.046100672,0.4084,0.2972,0.5323,0.1099,0.0934,0.0763,0.1516,0.1520,4.9349,0f000001,0*72236ee9\n\tsystem status\tnormal 2 27.800000 0 0\trobot status\t228.981497\t104.851041\t8.386100\t-1.313432\t0.996574\t-16.046101\t0.360000\t-0.048000\n\t\n15:19:48.8\tlog_raw\tgps_raw\t\tsystem status\tnormal 2 27.800000 0 0\trobot status\t229.109511\t104.803836\t8.392600\t-1.267387\t1.029682\t-15.166966\t0.241000\t0.102000\n\t\n15:19:49.3\tlog_raw\tgps_raw\t#INSPVAXA,USB3,0,49.0,FINESTEERING,2107,282007.350,02000000,471d,15824;INS_ALIGNMENT_COMPLETE,INS_RTKFIXED,37.37107412137,126.72342315241,8.3985,22.3000,-0.0946,0.2769,0.0276,-1.358512110,1.052240106,104.351657391,0.4091,0.2973,0.5323,0.1098,0.0932,0.0763,0.1515,0.1519,4.9361,0f000001,0*6aff20b9\n\tsystem status\tnormal 2 27.900000 0 0\trobot status\t229.244992\t104.757981\t8.398500\t-1.358512\t1.052240\t-14.351657\t0.380000\t-0.076000\n\t\n15:19:49.8\tlog_raw\tgps_raw\t\tsystem status\tnormal 2 27.900000 0 0\trobot status\t229.378040\t104.713852\t8.402400\t-1.303168\t1.125570\t-13.623239\t0.342000\t-0.051000\n\t\n15:19:50.3\tlog_raw\tgps_raw\t\tsystem status\tnormal 2 27.900000 0 0\trobot status\t229.513196\t104.672180\t8.406000\t-1.456812\t0.980332\t-13.050700\t0.312000\t-0.020000\n\t\n15:19:50.8\tlog_raw\tgps_raw\t\tsystem status\tnormal 2 28.000000 0 0\trobot status\t229.650581\t104.630716\t8.409400\t-1.501653\t0.682709\t-12.568671\t0.332000\t-0.055000\n\t\n15:19:51.3\tlog_raw\tgps_raw\t#INSPVAXA,USB3,0,47.0,FINESTEERING,2107,282009.350,02000000,471d,15824;INS_ALIGNMENT_COMPLETE,INS_RTKFIXED,37.37107260212,126.72342930936,8.4118,22.3000,-0.0884,0.2755,0.0223,-1.652819508,0.448050355,102.238648457,0.4104,0.2979,0.5346,0.1094,0.0930,0.0765,0.1512,0.1518,4.9380,0f000001,0*2e51505f\n\tsystem status\tnormal 2 28.000000 0 0\trobot status\t229.790365\t104.589353\t8.411800\t-1.652820\t0.448050\t-12.238648\t0.241000\t0.095000\n\t\n15:19:51.8\tlog_raw\tgps_raw\t#INSPVAXA,USB3,0,47.0,FINESTEERING,2107,282009.850,02000000,471d,15824;INS_ALIGNMENT_COMPLETE,INS_RTKFIXED,37.37107223648,126.72343083952,8.4130,22.3000,-0.0862,0.2839,0.0131,-1.656636551,0.434054933,102.188097613,0.4104,0.2979,0.5346,0.1094,0.0930,0.0765,0.1512,0.1518,4.9380,0f000001,0*992372f4\n\tsystem status\tnormal 2 28.000000 0 0\trobot status\t229.925904\t104.548769\t8.413000\t-1.656637\t0.434055\t-12.188098\t0.448000\t-0.230000\n\t\n15:19:52.3\tlog_raw\tgps_raw\t#INSPVAXA,USB3,0,46.0,FINESTEERING,2107,282010.350,02000000,471d,15824;INS_ALIGNMENT_COMPLETE,INS_RTKFIXED,37.37107186775,126.72343236378,8.4152,22.3000,-0.0921,0.2683,0.0190,-1.511067281,0.481994622,102.142666478,0.4105,0.2980,0.5358,0.1093,0.0929,0.0765,0.1512,0.1517,4.9389,0f000001,0*34dbbab6\n\tsystem status\tnormal 2 28.100000 0 0\trobot status\t230.060920\t104.507842\t8.415200\t-1.511067\t0.481995\t-12.142666\t0.265000\t0.040000\n\t\n15:19:52.8\tlog_raw\tgps_raw\t\tsystem status\tnormal 2 28.100000 0 0\trobot status\t230.195995\t104.467348\t8.417100\t-1.373778\t0.549233\t-12.226387\t0.303000\t-0.006000\n\t\n15:19:53.3\tlog_raw\tgps_raw\t#INSPVAXA,USB3,0,49.0,FINESTEERING,2107,282011.350,02000000,471d,15824;INS_ALIGNMENT_COMPLETE,INS_RTKFIXED,37.37107115288,126.72343536297,8.4170,22.3000,-0.0915,0.2655,0.0124,-1.290050138,0.612762474,102.317244842,0.4100,0.2979,0.5362,0.1091,0.0927,0.0765,0.1511,0.1517,4.9398,0f000001,0*277eff4c\n\tsystem status\tnormal 2 28.100000 0 0\trobot status\t230.326583\t104.428495\t8.417000\t-1.290050\t0.612762\t-12.317245\t0.295000\t-0.019000\n\t\n15:19:53.8\tlog_raw\tgps_raw\t\tsystem status\tnormal 2 28.100000 0 0\trobot status\t230.458276\t104.390451\t8.415800\t-1.393089\t0.652332\t-12.464453\t0.297000\t-0.032000\n\t\n15:19:54.3\tlog_raw\tgps_raw\t#INSPVAXA,USB3,0,48.5,FINESTEERING,2107,282012.350,02000000,471d,15824;INS_ALIGNMENT_COMPLETE,INS_RTKFIXED,37.37107045869,126.72343838460,8.4146,22.3000,-0.0891,0.2830,0.0038,-1.422267126,0.594621052,102.638304107,0.4097,0.2976,0.5361,0.1090,0.0927,0.0765,0.1511,0.1517,4.9408,0f000001,0*744e9f55\n\tsystem status\tnormal 2 28.100000 0 0\trobot status\t230.594234\t104.351443\t8.414600\t-1.422267\t0.594621\t-12.638304\t0.299000\t-0.028000\n\t\n15:19:54.8\tlog_raw\tgps_raw\t\tsystem status\tnormal 2 28.100000 0 0\trobot status\t230.727900\t104.312067\t8.415300\t-1.324093\t0.491707\t-12.894103\t0.295000\t-0.023000\n\t\n15:19:55.3\tlog_raw\tgps_raw\t\tsystem status\tnormal 2 28.100000 0 0\trobot status\t230.876200\t104.267210\t8.416800\t-1.101350\t0.506086\t-13.108771\t0.302000\t-0.022000\n\t\n15:19:55.8\tlog_raw\tgps_raw\t\tsystem status\tnormal 2 28.100000 0 0\trobot status\t231.020382\t104.222377\t8.418300\t-0.905486\t0.348570\t-13.416397\t0.226000\t-0.147000\n\t\n15:19:56.3\tlog_raw\tgps_raw\t\tsystem status\tnormal 2 28.000000 0 0\trobot status\t231.159139\t104.178286\t8.419100\t-0.919822\t0.431579\t-13.879981\t0.335000\t0.017000\n\t\n15:19:56.8\tlog_raw\tgps_raw\t\tsystem status\tnormal 2 28.000000 0 0\trobot status\t231.293510\t104.132233\t8.419000\t-0.825150\t0.562403\t-14.568254\t0.248000\t-0.110000\n\t\n15:19:57.3\tlog_raw\tgps_raw\t\tsystem status\tnormal 2 27.900000 0 0\trobot status\t231.430426\t104.084707\t8.419500\t-0.840035\t0.580522\t-15.437803\t0.249000\t-0.115000\n\t\n15:19:57.8\tlog_raw\tgps_raw\t#INSPVAXA,USB3,0,46.5,FINESTEERING,2107,282015.850,02000000,471d,15824;INS_ALIGNMENT_COMPLETE,INS_RTKFIXED,37.37106760969,126.72344937900,8.4187,22.3000,-0.0917,0.2780,0.0158,-0.823777305,0.513346415,106.387079923,0.4071,0.2967,0.5334,0.1088,0.0928,0.0762,0.1512,0.1516,4.9449,0f000001,0*de85c605\n\tsystem status\tnormal 2 27.900000 0 0\trobot status\t231.568100\t104.035221\t8.418700\t-0.823777\t0.513346\t-16.387080\t0.250000\t-0.115000\n\t\n15:19:58.3\tlog_raw\tgps_raw\t#INSPVAXA,USB3,0,46.0,FINESTEERING,2107,282016.350,02000000,471d,15824;INS_ALIGNMENT_COMPLETE,INS_RTKFIXED,37.37106713807,126.72345092537,8.4175,22.3000,-0.1003,0.2625,0.0249,-0.751765663,0.448430212,107.196344846,0.4062,0.2963,0.5317,0.1087,0.0929,0.0761,0.1512,0.1516,4.9459,0f000001,0*2521d5ac\n\tsystem status\tnormal 2 27.900000 0 0\trobot status\t231.705075\t103.982875\t8.417500\t-0.751766\t0.448430\t-17.196345\t0.230000\t-0.125000\n\t\n15:19:58.8\tlog_raw\tgps_raw\t#INSPVAXA,USB3,0,46.0,FINESTEERING,2107,282016.850,02000000,471d,15824;INS_ALIGNMENT_COMPLETE,INS_RTKFIXED,37.37106663656,126.72345246324,8.4162,22.3000,-0.1297,0.2604,0.0145,-0.574430267,0.261467814,108.063333899,0.4062,0.2963,0.5317,0.1087,0.0929,0.0761,0.1512,0.1516,4.9459,0f000001,0*0cb415b8\n\tsystem status\tnormal 2 27.900000 0 0\trobot status\t231.841297\t103.927211\t8.416200\t-0.574430\t0.261468\t-18.063334\t0.269000\t-0.057000\n\t\n15:19:59.3\tlog_raw\tgps_raw\t\tsystem status\tnormal 2 28.000000 0 0\trobot status\t231.975196\t103.870413\t8.415200\t-0.442412\t0.055156\t-19.022009\t0.322000\t0.000000\n\t\n15:19:59.8\tlog_raw\tgps_raw\t\tsystem status\tnormal 2 28.000000 0 0\trobot status\t232.108340\t103.813570\t8.414500\t-0.545377\t0.058818\t-19.694004\t0.288000\t-0.025000\n\t\n15:20:00.3\tlog_raw\tgps_raw\t\tsystem status\tnormal 2 28.000000 0 0\trobot status\t232.240742\t103.755119\t8.413400\t-0.645391\t0.147957\t-20.212329\t0.377000\t0.106000\n\t\n15:20:00.8\tlog_raw\tgps_raw\t\tsystem status\tnormal 2 28.000000 0 0\trobot status\t232.372937\t103.695535\t8.412700\t-0.738607\t0.123136\t-20.612001\t0.286000\t-0.029000\n\t\n15:20:01.3\tlog_raw\tgps_raw\t\tsystem status\tnormal 2 28.100000 0 0\trobot status\t232.504577\t103.633056\t8.410600\t-0.533313\t0.012430\t-20.893317\t0.309000\t0.005000\n\t\n15:20:01.8\tlog_raw\tgps_raw\t\tsystem status\tnormal 2 28.100000 0 0\trobot status\t232.631455\t103.572318\t8.407700\t-0.419591\t-0.044000\t-21.135314\t0.280000\t-0.004000\n\t\n15:20:02.3\tlog_raw\tgps_raw\t\tsystem status\tnormal 2 28.100000 0 0\trobot status\t232.760515\t103.510778\t8.407900\t-0.363601\t-0.080484\t-21.343355\t0.296000\t0.005000\n\t\n15:20:02.8\tlog_raw\tgps_raw\t\tsystem status\tnormal 2 28.100000 0 0\trobot status\t232.886836\t103.451179\t8.409100\t-0.420589\t-0.133663\t-21.544819\t0.302000\t0.006000\n\t\n15:20:03.3\tlog_raw\tgps_raw\t\tsystem status\tnormal 2 28.100000 0 0\trobot status\t233.012464\t103.392608\t8.407400\t-0.584557\t-0.078342\t-21.644193\t0.298000\t0.012000\n\t\n15:20:03.8\tlog_raw\tgps_raw\t\tsystem status\tnormal 2 28.100000 0 0\trobot status\t233.146755\t103.329041\t8.403700\t-0.539214\t0.104936\t-21.742041\t0.305000\t0.008000\n\t\n15:20:04.3\tlog_raw\tgps_raw\t\tsystem status\tnormal 2 28.100000 0 0\trobot status\t233.272452\t103.265686\t8.401800\t-0.266663\t0.108759\t-21.741358\t0.308000\t0.008000\n\t\n15:20:04.8\tlog_raw\tgps_raw\t\tsystem status\tnormal 2 28.100000 0 0\trobot status\t233.408317\t103.197854\t8.400500\t-0.012203\t-0.205668\t-21.761164\t0.313000\t0.000000\n\t\n15:20:05.4\tlog_raw\tgps_raw\t\tsystem status\tnormal 2 28.100000 0 0\trobot status\t233.537075\t103.135658\t8.399500\t-0.048898\t-0.274731\t-21.594046\t0.288000\t0.033000\n\t\n15:20:05.9\tlog_raw\tgps_raw\t\tsystem status\tnormal 2 28.000000 0 0\trobot status\t233.664757\t103.075029\t8.399500\t0.017553\t-0.318498\t-21.187224\t0.291000\t0.030000\n\t\n15:20:06.4\tlog_raw\tgps_raw\t\tsystem status\tnormal 2 27.900000 0 0\trobot status\t233.791563\t103.015014\t8.397500\t0.188872\t-0.337268\t-20.578425\t0.230000\t0.136000\n\t\n15:20:06.9\tlog_raw\tgps_raw\t\tsystem status\tnormal 
